vi "Process LIN Error Info Cluster.vi"(8 "Sprachliste":string[][](array[string]), 11 "Errors":T1) -> (2 "Störung":bool, 3 "String":string)   [LabVIEW 2020, in "Linearisierung v2.lvlib" / "SpanEinstellungen.lvlib"]
uses:
  SpanEinstellungen.lvlib
  LIN ErrorCluster.ctl
  Sprachverwaltung/Sprachverwaltung.lvlib
  Linearisierung v2.lvlib
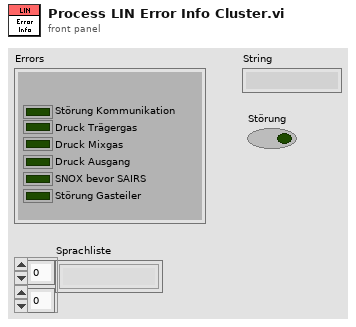
[diagram p1: front panel]
types:
  T1 = typedef "Linearisierung v2.lvlib/LIN ErrorCluster.ctl" = cluster{"Störung Kommunikation":bool, "Pressure carrier gas":bool, "Pressure diluted gas":bool, "Outlet Pressure":bool, "SNOX before SAIR":bool, "Störung Gasteiler":bool}
  T2 = cluster{"Label.Text":string, "Störung Kommunikation":bool}[]
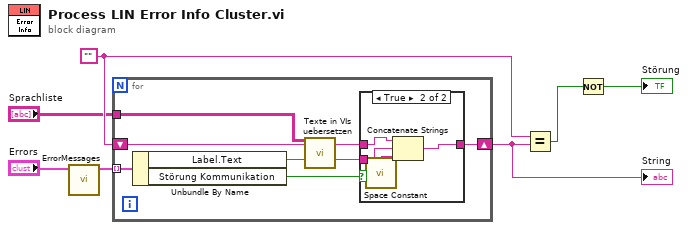
[diagram p0: block diagram]
diagram:
  w4 = ""
  n1 = call "ErrorMessages.vi"("Errors"="Errors") -> ("Error Array"=w5:T2)  [unwired: 9 in, 1 out]
  n2 = for {
    tunnel: w5 -> [w14] mode=indexing
    shift-right: [w12] -> w7
    shift-left: w4 -> [w11]
    tunnel: "Sprachliste" -> [w8]
    n3 = Unbundle By Name(w14) -> ("Label.Text"=w10:string, "Störung Kommunikation"=w13:bool)
    n4 = call "Texte in VIs uebersetzen.vi"("Sprachliste"=w8, "String zum Übersetzen"=w10) -> ("String zum Übersetzen"=w9:string)  [unwired: 9 in, 4 out]
    n5 = case shown="True" w13 {
      tunnel: w9 -> [_ w19]
      tunnel: [w15 w18] -> w12
      tunnel: w11 -> [w15 w16]
      frame False {
      }
      frame True {
        n6 = call <vilib>:"Space Constant.vi"() -> ("String"=w17:string)
        n7 = Concatenate Strings(w16, w19, w17) -> (w18:string)
      }
    }
  }
  "String" <- w7
  n8 = Equal?(x=w4, y=w7) -> (x = y?=w3:bool)
  n9 = Not(x=w3) -> (.not. x?=→"Störung":bool)
